vi "TCE_SaveConfiguration.vi"(0 "input cluster":T1={"Core"={"Current VI Reference"=refnum, "Close Panel on Exit?"=FALSE}, "Image Out"=refnum, "State"=0, "Points"={"Top Left"={"X"=0.0, "Y"=0.0}, "Top Right"={"X"=0.0, "Y"=0.0}, "Bottom Left"={"X"=0.0, "Y"=0.0}, "Bottom Right"={"X"=0.0, "Y"=0.0}, "x space 2"=0.0, "y space 2"=0.0, "x_space"=0.0, "y_space"=0.0, "Pixels"=[], "Fixpoint"={"X"=0.0, "Y"=0.0}}, "img_array"=[], "Temps"=[], "Temps_Array"=[], "Scan Area"=0.0, "Fixpoint Area"=0.0, "Config"={"Freezing"={"Cutoff"=2.0, "EndIndex"=2}}, "PCR Size"=0, "ImageCount"=0, "ShowGradient"=FALSE} {"Points"."Bottom Right"."Y" format="%.2f"; "Points"."Bottom Right"."X" format="%.2f"; "Points"."Top Left"."Y" format="%.2f"; "Points"."Top Left"."X" format="%.2f"; "Points"."Top Right"."Y" format="%.2f"; "Points"."Top Right"."X" format="%.2f"; "Points"."Bottom Left"."Y" format="%.2f"; "Points"."Bottom Left"."X" format="%.2f"; "Points"."Fixpoint"."Y" format="%.2f"; "Points"."Fixpoint"."X" format="%.2f"}, 1 "Temps":dbl[][](graph), 2 "FreezeTemps":dbl[](array[numeric]), 3 "MeltTemps":dbl[](array[numeric]), 4 "FrozenFraction":dbl[](array[numeric]), 5 "PartitionArray":string[](array[string]), 7 "Offsets":dbl[](array[numeric]), 9 "Offset Applied?":bool) -> (14 "Save Array out":string[][](array[string]), 17 "Full Array":string[][](array[string]), 19 "Canceled":bool)   [LabVIEW 2022 SP3]
uses:
  DataCluster_TCAL.ctl
  <vilib>/vision/Image Controls.llb/IMAQ Image.ctl
  TCE_Config.ctl
panel:
  in  "Nm(T)":bool=TRUE
  in  "SaveFrozen":bool=TRUE caption="Frozen Fraction"
  in  "SaveMelt":bool=TRUE caption="Melting Point"
  in  "SaveFreeze":bool=TRUE caption="Freezing Point"
  in  "SaveTemp":bool=TRUE caption="Temperatures"
  out "Data Array":string[][](array[string])=[["Well Name", "Content", "Freeze Temp", "Melting Temp", "T0..."], ["Calibration Offset", "Not Applied", "", "", ""], ["A1", "", "", "", ""], ["B1", "", "", "", ""], ["C1", "", "", "", ""], ["D1", "", "", "", ""], ["E1", "", "", "", ""], ["F1", "", "", "", ""], ["G1", "", "", "", ""], ["H1", "", "", "", ""], ["I1", "", "", "", ""], ["J1", "", "", "", ""], ["K1", "", "", "", ""], ["L1", "", "", "", ""], ["M1", "", "", "", ""], ["N1", "", "", "", ""], ["O1", "", "", "", ""], ["P1", "", "", "", ""], ["A2", "", "", "", ""], ["B2", "", "", "", ""], ["C2", "", "", "", ""], ["D2", "", "", "", ""], ["E2", "", "", "", ""], ["F2", "", "", "", ""], ["G2", "", "", "", ""], ["H2", "", "", "", ""], ["I2", "", "", "", ""], ["J2", "", "", "", ""], ["K2", "", "", "", ""], ["L2", "", "", "", ""], ["M2", "", "", "", ""], ["N2", "", "", "", ""], ["O2", "", "", "", ""], ["P2", "", "", "", ""], ["A3", "", "", "", ""], ["B3", "", "", "", ""], ["C3", "", "", "", ""], ["D3", "", "", "", ""], ["E3", "", "", "", ""], ["F3", "", "", "", ""], ["G3", "", "", "", ""], ["H3", "", "", "", ""], ["I3", "", "", "", ""], ["J3", "", "", "", ""], ["K3", "", "", "", ""], ["L3", "", "", "", ""], ["M3", "", "", "", ""], ["N3", "", "", "", ""], ["O3", "", "", "", ""], ["P3", "", "", "", ""], ["A4", "", "", "", ""], ["B4", "", "", "", ""], ["C4", "", "", "", ""], ["D4", "", "", "", ""], ["E4", "", "", "", ""], ["F4", "", "", "", ""], ["G4", "", "", "", ""], ["H4", "", "", "", ""], ["I4", "", "", "", ""], ["J4", "", "", "", ""], ["K4", "", "", "", ""], ["L4", "", "", "", ""], ["M4", "", "", "", ""], ["N4", "", "", "", ""], ["O4", "", "", "", ""], ["P4", "", "", "", ""], ["A5", "", "", "", ""], ["B5", "", "", "", ""], ["C5", "", "", "", ""], ["D5", "", "", "", ""], ["E5", "", "", "", ""], ["F5", "", "", "", ""], ["G5", "", "", "", ""], ["H5", "", "", "", ""], ["I5", "", "", "", ""], ["J5", "", "", "", ""], ["K5", "", "", "", ""], ["L5", "", "", "", ""], ["M5", "", "", "", ""], ["N5", "", "", "", ""], ["O5", "", "", "", ""], ["P5", "", "", "", ""], ["A6", "", "", "", ""], ["B6", "", "", "", ""], ["C6", "", "", "", ""], ["D6", "", "", "", ""], ["E6", "", "", "", ""], ["F6", "", "", "", ""], ["G6", "", "", "", ""], ["H6", "", "", "", ""], ["I6", "", "", "", ""], ["J6", "", "", "", ""], ["K6", "", "", "", ""], ["L6", "", "", "", ""], ["M6", "", "", "", ""], ["N6", "", "", "", ""], ["O6", "", "", "", ""], ["P6", "", "", "", ""], ["A7", "", "", "", ""], ["B7", "", "", "", ""], ["C7", "", "", "", ""], ["D7", "", "", "", ""], ["E7", "", "", "", ""], ["F7", "", "", "", ""], ["G7", "", "", "", ""], ["H7", "", "", "", ""], ["I7", "", "", "", ""], ["J7", "", "", "", ""], ["K7", "", "", "", ""], ["L7", "", "", "", ""], ["M7", "", "", "", ""], ["N7", "", "", "", ""], ["O7", "", "", "", ""], ["P7", "", "", "", ""], ["A8", "", "", "", ""], ["B8", "", "", "", ""], ["C8", "", "", "", ""], ["D8", "", "", "", ""], ["E8", "", "", "", ""], ["F8", "", "", "", ""], ["G8", "", "", "", ""], ["H8", "", "", "", ""], ["I8", "", "", "", ""], ["J8", "", "", "", ""], ["K8", "", "", "", ""], ["L8", "", "", "", ""], ["M8", "", "", "", ""], ["N8", "", "", "", ""], ["O8", "", "", "", ""], ["P8", "", "", "", ""], ["A9", "", "", "", ""], ["B9", "", "", "", ""], ["C9", "", "", "", ""], ["D9", "", "", "", ""], ["E9", "", "", "", ""], ["F9", "", "", "", ""], ["G9", "", "", "", ""], ["H9", "", "", "", ""], ["I9", "", "", "", ""], ["J9", "", "", "", ""], ["K9", "", "", "", ""], ["L9", "", "", "", ""], ["M9", "", "", "", ""], ["N9", "", "", "", ""], ["O9", "", "", "", ""], ["P9", "", "", "", ""], ["A10", "", "", "", ""], ["B10", "", "", "", ""], ["C10", "", "", "", ""], ["D10", "", "", "", ""], ["E10", "", "", "", ""], ["F10", "", "", "", ""], ["G10", "", "", "", ""], ["H10", "", "", "", ""], ["I10", "", "", "", ""], ["J10", "", "", "", ""], ["K10", "", "", "", ""], ["L10", "", "", "", ""], ["M10", "", "", "", ""], ["N10", "", "", "", ""], ["O10", "", "", "", ""], ["P10", "", "", "", ""], ["A11", "", "", "", ""], ["B11", "", "", "", ""], ["C11", "", "", "", ""], ["D11", "", "", "", ""], ["E11", "", "", "", ""], ["F11", "", "", "", ""], ["G11", "", "", "", ""], ["H11", "", "", "", ""], ["I11", "", "", "", ""], ["J11", "", "", "", ""], ["K11", "", "", "", ""], ["L11", "", "", "", ""], ["M11", "", "", "", ""], ["N11", "", "", "", ""], ["O11", "", "", "", ""], ["P11", "", "", "", ""], ["A12", "", "", "", ""], ["B12", "", "", "", ""], ["C12", "", "", "", ""], ["D12", "", "", "", ""], ["E12", "", "", "", ""], ["F12", "", "", "", ""], ["G12", "", "", "", ""], ["H12", "", "", "", ""], ["I12", "", "", "", ""], ["J12", "", "", "", ""], ["K12", "", "", "", ""], ["L12", "", "", "", ""], ["M12", "", "", "", ""], ["N12", "", "", "", ""], ["O12", "", "", "", ""], ["P12", "", "", "", ""], ["A13", "", "", "", ""], ["B13", "", "", "", ""], ["C13", "", "", "", ""], ["D13", "", "", "", ""], ["E13", "", "", "", ""], ["F13", "", "", "", ""], ["G13", "", "", "", ""], ["H13", "", "", "", ""], ["I13", "", "", "", ""], ["J13", "", "", "", ""], ["K13", "", "", "", ""], ["L13", "", "", "", ""], ["M13", "", "", "", ""], ["N13", "", "", "", ""], ["O13", "", "", "", ""], ["P13", "", "", "", ""], ["A14", "", "", "", ""], ["B14", "", "", "", ""], ["C14", "", "", "", ""], ["D14", "", "", "", ""], ["E14", "", "", "", ""], ["F14", "", "", "", ""], ["G14", "", "", "", ""], ["H14", "", "", "", ""], ["I14", "", "", "", ""], ["J14", "", "", "", ""], ["K14", "", "", "", ""], ["L14", "", "", "", ""], ["M14", "", "", "", ""], ["N14", "", "", "", ""], ["O14", "", "", "", ""], ["P14", "", "", "", ""], ["A15", "", "", "", ""], ["B15", "", "", "", ""], ["C15", "", "", "", ""], ["D15", "", "", "", ""], ["E15", "", "", "", ""], ["F15", "", "", "", ""], ["G15", "", "", "", ""], ["H15", "", "", "", ""], ["I15", "", "", "", ""], ["J15", "", "", "", ""], ["K15", "", "", "", ""], ["L15", "", "", "", ""], ["M15", "", "", "", ""], ["N15", "", "", "", ""], ["O15", "", "", "", ""], ["P15", "", "", "", ""], ["A16", "", "", "", ""], ["B16", "", "", "", ""], ["C16", "", "", "", ""], ["D16", "", "", "", ""], ["E16", "", "", "", ""], ["F16", "", "", "", ""], ["G16", "", "", "", ""], ["H16", "", "", "", ""], ["I16", "", "", "", ""], ["J16", "", "", "", ""], ["K16", "", "", "", ""], ["L16", "", "", "", ""], ["M16", "", "", "", ""], ["N16", "", "", "", ""], ["O16", "", "", "", ""], ["P16", "", "", "", ""], ["A17", "", "", "", ""], ["B17", "", "", "", ""], ["C17", "", "", "", ""], ["D17", "", "", "", ""], ["E17", "", "", "", ""], ["F17", "", "", "", ""], ["G17", "", "", "", ""], ["H17", "", "", "", ""], ["I17", "", "", "", ""], ["J17", "", "", "", ""], ["K17", "", "", "", ""], ["L17", "", "", "", ""], ["M17", "", "", "", ""], ["N17", "", "", "", ""], ["O17", "", "", "", ""], ["P17", "", "", "", ""], ["A18", "", "", "", ""], ["B18", "", "", "", ""], ["C18", "", "", "", ""], ["D18", "", "", "", ""], ["E18", "", "", "", ""], ["F18", "", "", "", ""], ["G18", "", "", "", ""], ["H18", "", "", "", ""], ["I18", "", "", "", ""], ["J18", "", "", "", ""], ["K18", "", "", "", ""], ["L18", "", "", "", ""], ["M18", "", "", "", ""], ["N18", "", "", "", ""], ["O18", "", "", "", ""], ["P18", "", "", "", ""], ["A19", "", "", "", ""], ["B19", "", "", "", ""], ["C19", "", "", "", ""], ["D19", "", "", "", ""], ["E19", "", "", "", ""], ["F19", "", "", "", ""], ["G19", "", "", "", ""], ["H19", "", "", "", ""], ["I19", "", "", "", ""], ["J19", "", "", "", ""], ["K19", "", "", "", ""], ["L19", "", "", "", ""], ["M19", "", "", "", ""], ["N19", "", "", "", ""], ["O19", "", "", "", ""], ["P19", "", "", "", ""], ["A20", "", "", "", ""], ["B20", "", "", "", ""], ["C20", "", "", "", ""], ["D20", "", "", "", ""], ["E20", "", "", "", ""], ["F20", "", "", "", ""], ["G20", "", "", "", ""], ["H20", "", "", "", ""], ["I20", "", "", "", ""], ["J20", "", "", "", ""], ["K20", "", "", "", ""], ["L20", "", "", "", ""], ["M20", "", "", "", ""], ["N20", "", "", "", ""], ["O20", "", "", "", ""], ["P20", "", "", "", ""], ["A21", "", "", "", ""], ["B21", "", "", "", ""], ["C21", "", "", "", ""], ["D21", "", "", "", ""], ["E21", "", "", "", ""], ["F21", "", "", "", ""], ["G21", "", "", "", ""], ["H21", "", "", "", ""], ["I21", "", "", "", ""], ["J21", "", "", "", ""], ["K21", "", "", "", ""], ["L21", "", "", "", ""], ["M21", "", "", "", ""], ["N21", "", "", "", ""], ["O21", "", "", "", ""], ["P21", "", "", "", ""], ["A22", "", "", "", ""], ["B22", "", "", "", ""], ["C22", "", "", "", ""], ["D22", "", "", "", ""], ["E22", "", "", "", ""], ["F22", "", "", "", ""], ["G22", "", "", "", ""], ["H22", "", "", "", ""], ["I22", "", "", "", ""], ["J22", "", "", "", ""], ["K22", "", "", "", ""], ["L22", "", "", "", ""], ["M22", "", "", "", ""], ["N22", "", "", "", ""], ["O22", "", "", "", ""], ["P22", "", "", "", ""], ["A23", "", "", "", ""], ["B23", "", "", "", ""], ["C23", "", "", "", ""], ["D23", "", "", "", ""], ["E23", "", "", "", ""], ["F23", "", "", "", ""], ["G23", "", "", "", ""], ["H23", "", "", "", ""], ["I23", "", "", "", ""], ["J23", "", "", "", ""], ["K23", "", "", "", ""], ["L23", "", "", "", ""], ["M23", "", "", "", ""], ["N23", "", "", "", ""], ["O23", "", "", "", ""], ["P23", "", "", "", ""], ["A24", "", "", "", ""], ["B24", "", "", "", ""], ["C24", "", "", "", ""], ["D24", "", "", "", ""], ["E24", "", "", "", ""], ["F24", "", "", "", ""], ["G24", "", "", "", ""], ["H24", "", "", "", ""], ["I24", "", "", "", ""], ["J24", "", "", "", ""], ["K24", "", "", "", ""], ["L24", "", "", "", ""], ["M24", "", "", "", ""], ["N24", "", "", "", ""], ["O24", "", "", "", ""], ["P24", "", "", "", ""]]
  in  "Cancel":bool
  in  "OK":bool
  # "Settings"
  # "File Preview"
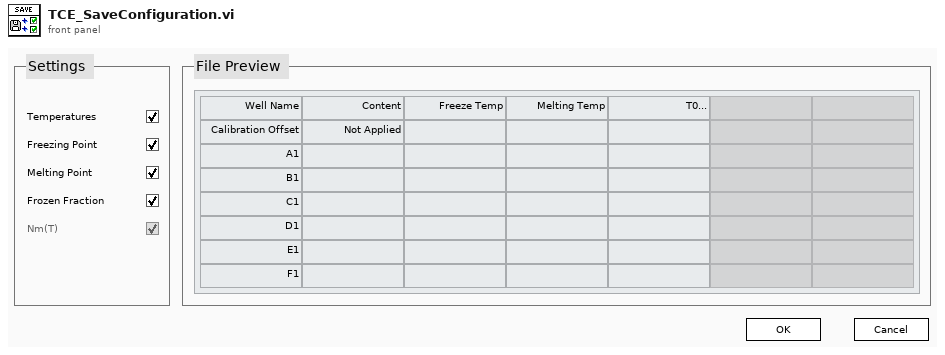
[diagram p1: front panel]
types:
  T1 = typedef "DataCluster_TCAL.ctl" = cluster{"Core":cluster{"Current VI Reference":refnum<vi>, "Close Panel on Exit?":bool}, "Image Out":T2, "State":i32, "Points":cluster{"Top Left":T3, "Top Right":T3, "Bottom Left":T3, "Bottom Right":T3, "x space 2":dbl, "y space 2":sgl, "x_space":sgl, "y_space":sgl, "Pixels":cluster{"X":i32, "Y":i32}[][], "Fixpoint":T3}, "img_array":T2[], "Temps":dbl[], "Temps_Array":dbl[][], "Scan Area":dbl, "Fixpoint Area":dbl, "Config":T4, "PCR Size":u16, "ImageCount":i32, "ShowGradient":bool}
  T2 = typedef "IMAQ Image.ctl" = refnum<image>
  T3 = typedef "IMAQ Point" = cluster{"X":sgl, "Y":sgl}
  T4 = typedef "TCE_Config.ctl" = cluster{"Freezing":cluster{"Cutoff":dbl, "EndIndex":i32}}
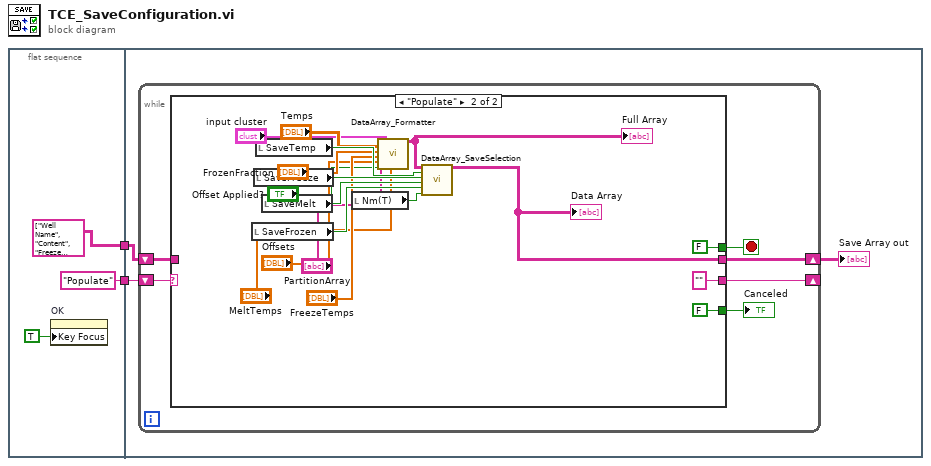
[diagram p0: block diagram]
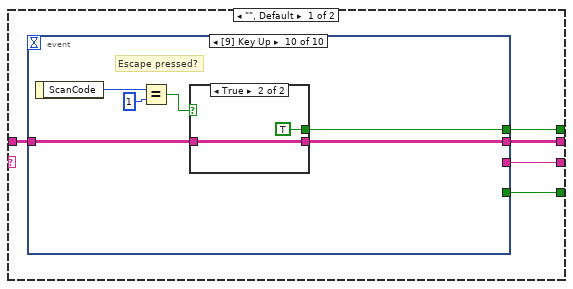
[diagram p2: hidden frame]
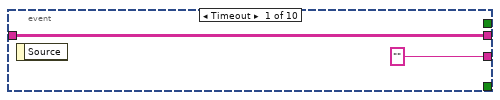
[diagram p3: hidden frame]
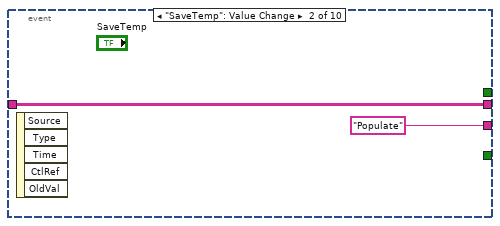
[diagram p4: hidden frame]
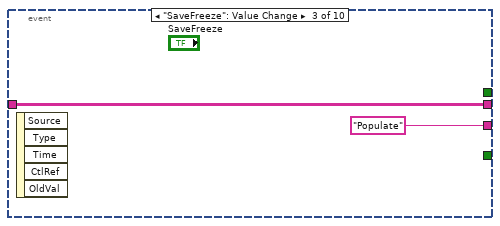
[diagram p5: hidden frame]
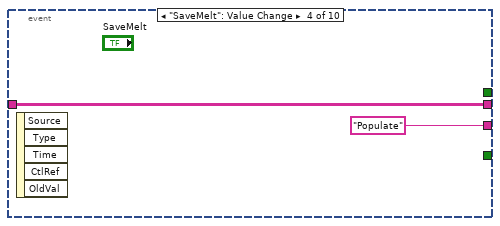
[diagram p6: hidden frame]
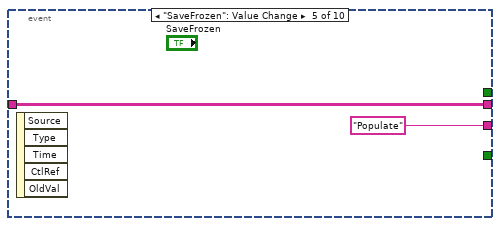
[diagram p7: hidden frame]
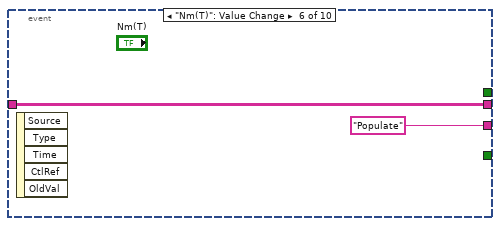
[diagram p8: hidden frame]
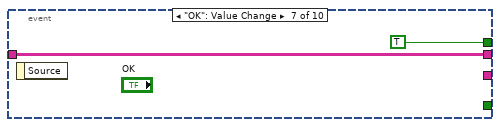
[diagram p9: hidden frame]
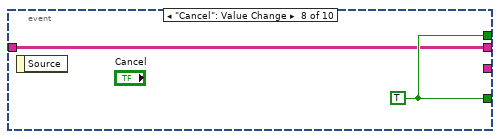
[diagram p10: hidden frame]
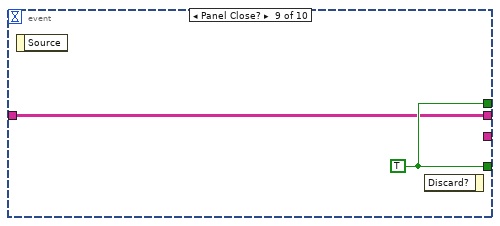
[diagram p11: hidden frame]
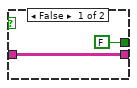
[diagram p12: hidden frame]
diagram:
  n1 = flat-sequence {
    tunnel: [string[][] [["Well Name", "Content", "Freeze Temp", "Melting Temp", "T0..."], ["Calibration Offset", "Not Applied", "", "", ""], ["A1", "", "", "", ""], ["B1", "", "", "", ""], ["C1", "", "", "", ""], ["D1", "", "", "", ""], ["E1", "", "", "", ""], ["F1", "", "", "", ""], ["G1", "", "", "", ""], ["H1", "", "", "", ""], ["I1", "", "", "", ""], ["J1", "", "", "", ""], ["K1", "", "", "", ""], ["L1", "", "", "", ""], ["M1", "", "", "", ""], ["N1", "", "", "", ""], ["O1", "", "", "", ""], ["P1", "", "", "", ""], ["A2", "", "", "", ""], ["B2", "", "", "", ""], ["C2", "", "", "", ""], ["D2", "", "", "", ""], ["E2", "", "", "", ""], ["F2", "", "", "", ""], ["G2", "", "", "", ""], ["H2", "", "", "", ""], ["I2", "", "", "", ""], ["J2", "", "", "", ""], ["K2", "", "", "", ""], ["L2", "", "", "", ""], ["M2", "", "", "", ""], ["N2", "", "", "", ""], ["O2", "", "", "", ""], ["P2", "", "", "", ""], ["A3", "", "", "", ""], ["B3", "", "", "", ""], ["C3", "", "", "", ""], ["D3", "", "", "", ""], ["E3", "", "", "", ""], ["F3", "", "", "", ""], ["G3", "", "", "", ""], ["H3", "", "", "", ""], ["I3", "", "", "", ""], ["J3", "", "", "", ""], ["K3", "", "", "", ""], ["L3", "", "", "", ""], ["M3", "", "", "", ""], ["N3", "", "", "", ""], ["O3", "", "", "", ""], ["P3", "", "", "", ""], ["A4", "", "", "", ""], ["B4", "", "", "", ""], ["C4", "", "", "", ""], ["D4", "", "", "", ""], ["E4", "", "", "", ""], ["F4", "", "", "", ""], ["G4", "", "", "", ""], ["H4", "", "", "", ""], ["I4", "", "", "", ""], ["J4", "", "", "", ""], ["K4", "", "", "", ""], ["L4", "", "", "", ""], ["M4", "", "", "", ""], ["N4", "", "", "", ""], ["O4", "", "", "", ""], ["P4", "", "", "", ""], ["A5", "", "", "", ""], ["B5", "", "", "", ""], ["C5", "", "", "", ""], ["D5", "", "", "", ""], ["E5", "", "", "", ""], ["F5", "", "", "", ""], ["G5", "", "", "", ""], ["H5", "", "", "", ""], ["I5", "", "", "", ""], ["J5", "", "", "", ""], ["K5", "", "", "", ""], ["L5", "", "", "", ""], ["M5", "", "", "", ""], ["N5", "", "", "", ""], ["O5", "", "", "", ""], ["P5", "", "", "", ""], ["A6", "", "", "", ""], ["B6", "", "", "", ""], ["C6", "", "", "", ""], ["D6", "", "", "", ""], ["E6", "", "", "", ""], ["F6", "", "", "", ""], ["G6", "", "", "", ""], ["H6", "", "", "", ""], ["I6", "", "", "", ""], ["J6", "", "", "", ""], ["K6", "", "", "", ""], ["L6", "", "", "", ""], ["M6", "", "", "", ""], ["N6", "", "", "", ""], ["O6", "", "", "", ""], ["P6", "", "", "", ""], ["A7", "", "", "", ""], ["B7", "", "", "", ""], ["C7", "", "", "", ""], ["D7", "", "", "", ""], ["E7", "", "", "", ""], ["F7", "", "", "", ""], ["G7", "", "", "", ""], ["H7", "", "", "", ""], ["I7", "", "", "", ""], ["J7", "", "", "", ""], ["K7", "", "", "", ""], ["L7", "", "", "", ""], ["M7", "", "", "", ""], ["N7", "", "", "", ""], ["O7", "", "", "", ""], ["P7", "", "", "", ""], ["A8", "", "", "", ""], ["B8", "", "", "", ""], ["C8", "", "", "", ""], ["D8", "", "", "", ""], ["E8", "", "", "", ""], ["F8", "", "", "", ""], ["G8", "", "", "", ""], ["H8", "", "", "", ""], ["I8", "", "", "", ""], ["J8", "", "", "", ""], ["K8", "", "", "", ""], ["L8", "", "", "", ""], ["M8", "", "", "", ""], ["N8", "", "", "", ""], ["O8", "", "", "", ""], ["P8", "", "", "", ""], ["A9", "", "", "", ""], ["B9", "", "", "", ""], ["C9", "", "", "", ""], ["D9", "", "", "", ""], ["E9", "", "", "", ""], ["F9", "", "", "", ""], ["G9", "", "", "", ""], ["H9", "", "", "", ""], ["I9", "", "", "", ""], ["J9", "", "", "", ""], ["K9", "", "", "", ""], ["L9", "", "", "", ""], ["M9", "", "", "", ""], ["N9", "", "", "", ""], ["O9", "", "", "", ""], ["P9", "", "", "", ""], ["A10", "", "", "", ""], ["B10", "", "", "", ""], ["C10", "", "", "", ""], ["D10", "", "", "", ""], ["E10", "", "", "", ""], ["F10", "", "", "", ""], ["G10", "", "", "", ""], ["H10", "", "", "", ""], ["I10", "", "", "", ""], ["J10", "", "", "", ""], ["K10", "", "", "", ""], ["L10", "", "", "", ""], ["M10", "", "", "", ""], ["N10", "", "", "", ""], ["O10", "", "", "", ""], ["P10", "", "", "", ""], ["A11", "", "", "", ""], ["B11", "", "", "", ""], ["C11", "", "", "", ""], ["D11", "", "", "", ""], ["E11", "", "", "", ""], ["F11", "", "", "", ""], ["G11", "", "", "", ""], ["H11", "", "", "", ""], ["I11", "", "", "", ""], ["J11", "", "", "", ""], ["K11", "", "", "", ""], ["L11", "", "", "", ""], ["M11", "", "", "", ""], ["N11", "", "", "", ""], ["O11", "", "", "", ""], ["P11", "", "", "", ""], ["A12", "", "", "", ""], ["B12", "", "", "", ""], ["C12", "", "", "", ""], ["D12", "", "", "", ""], ["E12", "", "", "", ""], ["F12", "", "", "", ""], ["G12", "", "", "", ""], ["H12", "", "", "", ""], ["I12", "", "", "", ""], ["J12", "", "", "", ""], ["K12", "", "", "", ""], ["L12", "", "", "", ""], ["M12", "", "", "", ""], ["N12", "", "", "", ""], ["O12", "", "", "", ""], ["P12", "", "", "", ""], ["A13", "", "", "", ""], ["B13", "", "", "", ""], ["C13", "", "", "", ""], ["D13", "", "", "", ""], ["E13", "", "", "", ""], ["F13", "", "", "", ""], ["G13", "", "", "", ""], ["H13", "", "", "", ""], ["I13", "", "", "", ""], ["J13", "", "", "", ""], ["K13", "", "", "", ""], ["L13", "", "", "", ""], ["M13", "", "", "", ""], ["N13", "", "", "", ""], ["O13", "", "", "", ""], ["P13", "", "", "", ""], ["A14", "", "", "", ""], ["B14", "", "", "", ""], ["C14", "", "", "", ""], ["D14", "", "", "", ""], ["E14", "", "", "", ""], ["F14", "", "", "", ""], ["G14", "", "", "", ""], ["H14", "", "", "", ""], ["I14", "", "", "", ""], ["J14", "", "", "", ""], ["K14", "", "", "", ""], ["L14", "", "", "", ""], ["M14", "", "", "", ""], ["N14", "", "", "", ""], ["O14", "", "", "", ""], ["P14", "", "", "", ""], ["A15", "", "", "", ""], ["B15", "", "", "", ""], ["C15", "", "", "", ""], ["D15", "", "", "", ""], ["E15", "", "", "", ""], ["F15", "", "", "", ""], ["G15", "", "", "", ""], ["H15", "", "", "", ""], ["I15", "", "", "", ""], ["J15", "", "", "", ""], ["K15", "", "", "", ""], ["L15", "", "", "", ""], ["M15", "", "", "", ""], ["N15", "", "", "", ""], ["O15", "", "", "", ""], ["P15", "", "", "", ""], ["A16", "", "", "", ""], ["B16", "", "", "", ""], ["C16", "", "", "", ""], ["D16", "", "", "", ""], ["E16", "", "", "", ""], ["F16", "", "", "", ""], ["G16", "", "", "", ""], ["H16", "", "", "", ""], ["I16", "", "", "", ""], ["J16", "", "", "", ""], ["K16", "", "", "", ""], ["L16", "", "", "", ""], ["M16", "", "", "", ""], ["N16", "", "", "", ""], ["O16", "", "", "", ""], ["P16", "", "", "", ""], ["A17", "", "", "", ""], ["B17", "", "", "", ""], ["C17", "", "", "", ""], ["D17", "", "", "", ""], ["E17", "", "", "", ""], ["F17", "", "", "", ""], ["G17", "", "", "", ""], ["H17", "", "", "", ""], ["I17", "", "", "", ""], ["J17", "", "", "", ""], ["K17", "", "", "", ""], ["L17", "", "", "", ""], ["M17", "", "", "", ""], ["N17", "", "", "", ""], ["O17", "", "", "", ""], ["P17", "", "", "", ""], ["A18", "", "", "", ""], ["B18", "", "", "", ""], ["C18", "", "", "", ""], ["D18", "", "", "", ""], ["E18", "", "", "", ""], ["F18", "", "", "", ""], ["G18", "", "", "", ""], ["H18", "", "", "", ""], ["I18", "", "", "", ""], ["J18", "", "", "", ""], ["K18", "", "", "", ""], ["L18", "", "", "", ""], ["M18", "", "", "", ""], ["N18", "", "", "", ""], ["O18", "", "", "", ""], ["P18", "", "", "", ""], ["A19", "", "", "", ""], ["B19", "", "", "", ""], ["C19", "", "", "", ""], ["D19", "", "", "", ""], ["E19", "", "", "", ""], ["F19", "", "", "", ""], ["G19", "", "", "", ""], ["H19", "", "", "", ""], ["I19", "", "", "", ""], ["J19", "", "", "", ""], ["K19", "", "", "", ""], ["L19", "", "", "", ""], ["M19", "", "", "", ""], ["N19", "", "", "", ""], ["O19", "", "", "", ""], ["P19", "", "", "", ""], ["A20", "", "", "", ""], ["B20", "", "", "", ""], ["C20", "", "", "", ""], ["D20", "", "", "", ""], ["E20", "", "", "", ""], ["F20", "", "", "", ""], ["G20", "", "", "", ""], ["H20", "", "", "", ""], ["I20", "", "", "", ""], ["J20", "", "", "", ""], ["K20", "", "", "", ""], ["L20", "", "", "", ""], ["M20", "", "", "", ""], ["N20", "", "", "", ""], ["O20", "", "", "", ""], ["P20", "", "", "", ""], ["A21", "", "", "", ""], ["B21", "", "", "", ""], ["C21", "", "", "", ""], ["D21", "", "", "", ""], ["E21", "", "", "", ""], ["F21", "", "", "", ""], ["G21", "", "", "", ""], ["H21", "", "", "", ""], ["I21", "", "", "", ""], ["J21", "", "", "", ""], ["K21", "", "", "", ""], ["L21", "", "", "", ""], ["M21", "", "", "", ""], ["N21", "", "", "", ""], ["O21", "", "", "", ""], ["P21", "", "", "", ""], ["A22", "", "", "", ""], ["B22", "", "", "", ""], ["C22", "", "", "", ""], ["D22", "", "", "", ""], ["E22", "", "", "", ""], ["F22", "", "", "", ""], ["G22", "", "", "", ""], ["H22", "", "", "", ""], ["I22", "", "", "", ""], ["J22", "", "", "", ""], ["K22", "", "", "", ""], ["L22", "", "", "", ""], ["M22", "", "", "", ""], ["N22", "", "", "", ""], ["O22", "", "", "", ""], ["P22", "", "", "", ""], ["A23", "", "", "", ""], ["B23", "", "", "", ""], ["C23", "", "", "", ""], ["D23", "", "", "", ""], ["E23", "", "", "", ""], ["F23", "", "", "", ""], ["G23", "", "", "", ""], ["H23", "", "", "", ""], ["I23", "", "", "", ""], ["J23", "", "", "", ""], ["K23", "", "", "", ""], ["L23", "", "", "", ""], ["M23", "", "", "", ""], ["N23", "", "", "", ""], ["O23", "", "", "", ""], ["P23", "", "", "", ""], ["A24", "", "", "", ""], ["B24", "", "", "", ""], ["C24", "", "", "", ""], ["D24", "", "", "", ""], ["E24", "", "", "", ""], ["F24", "", "", "", ""], ["G24", "", "", "", ""], ["H24", "", "", "", ""], ["I24", "", "", "", ""], ["J24", "", "", "", ""], ["K24", "", "", "", ""], ["L24", "", "", "", ""], ["M24", "", "", "", ""], ["N24", "", "", "", ""], ["O24", "", "", "", ""], ["P24", "", "", "", ""]] ("Data Array out")] -> w2
    tunnel: ["Populate"] -> w1
    tunnel: w2 -> [w8]
    tunnel: w1 -> [w7]
    frame #0 {
      n2 = property on="OK" class="Bool"("Key Focus"=TRUE) -> ()  [unwired: 2 in, 2 out]
    }
    frame #1 {
      n3 = while {
        shift-right: [w14] -> w6
        shift-left: w8 -> [w13]
        shift-right: [w9] -> _
        shift-left: w7 -> [w10]
        stop <- w12 stop-if-true
        n4 = case shown="\"Populate\"" w10 {
          tunnel: [w19 w48] -> w14
          tunnel: w13 -> [w18 _]
          tunnel: [w17 FALSE] -> w12
          tunnel: [w16 FALSE] -> w11
          tunnel: [w15 ""] -> w9
          frame "", Default {
            n5 = event shown="[9] Key Up" {
              selector: _ -> [_ _ _ _ _ _ _ _ _ _]
              dyn-events: _ -> [_ _ _ _ _ _ _ _ _ _]
              timeout: _ -> [_ _ _ _ _ _ _ _ _ _]
              tunnel: w18 -> [w20 w22 w24 w26 w28 w30 w33 w34 w36 w38]
              tunnel: [w20 w22 w24 w26 w28 w30 w33 w34 w36 w39] -> w19
              tunnel: [_ _ _ _ _ _ TRUE w35 w37 w43] -> w17
              tunnel: [_ _ _ _ _ _ _ w35 w37 _] -> w16
              tunnel: ["" "Populate" "Populate" "Populate" "Populate" "Populate" _ _ _ _] -> w15
              event Timeout {
                n6 = event-data() -> ()  [unwired: 1 in, 1 out]
              }
              event "SaveTemp": Value Change {
                n7 = event-data() -> ()  [unwired: 1 in, 5 out]
              }
              event "SaveFreeze": Value Change {
                n8 = event-data() -> ()  [unwired: 1 in, 5 out]
              }
              event "SaveMelt": Value Change {
                n9 = event-data() -> ()  [unwired: 1 in, 5 out]
              }
              event "SaveFrozen": Value Change {
                n10 = event-data() -> ()  [unwired: 1 in, 5 out]
              }
              event "Nm(T)": Value Change {
                n11 = event-data() -> ()  [unwired: 1 in, 5 out]
              }
              event "OK": Value Change {
                n12 = event-data() -> ()  [unwired: 1 in, 1 out]
              }
              event "Cancel": Value Change {
                w35 = TRUE
                n13 = event-data() -> ()  [unwired: 1 in, 1 out]
              }
              event Panel Close? {
                w37 = TRUE
                n14 = event-data() -> ()  [unwired: 1 in, 1 out]
                n15 = event-data() -> ()  [unwired: 2 in, 1 out]
              }
              event Key Up {
                # "Escape pressed?"
                n16 = event-data() -> ("ScanCode"=w42:i16)  [unwired: 1 in]
                n17 = Equal?(x=w42, y=i16 1) -> (x = y?=w40:bool)
                n18 = case shown="True" w40 {
                  tunnel: [FALSE TRUE] -> w43
                  tunnel: [w45 w46] -> w39
                  tunnel: w38 -> [w45 w46]
                  frame False {
                  }
                  frame True {
                  }
                }
              }
            }
          }
          frame "Populate" {
            n19 = local read "SaveFrozen"() -> (w59:bool)
            n20 = local read "SaveFreeze"() -> (w57:bool)
            n21 = local read "SaveTemp"() -> (w61:bool)
            n22 = local read "SaveMelt"() -> (w58:bool)
            n23 = local read "Nm(T)"() -> (w60:bool)
            n24 = call "DataArray_Formatter.vi"("PartitionArray"="PartitionArray", "Temps"="Temps", "FrozenFraction"="FrozenFraction", "FreezeTemps"="FreezeTemps", "Offsets"="Offsets", "Offset Applied?"="Offset Applied?", "input cluster"="input cluster", "MeltTemps"="MeltTemps") -> ("Data Array"=w62:string[][])  [unwired: 11 in]
            "Full Array" <- w62
            n25 = call "DataArray_SaveSelection.vi"("Data Array"=w62, "SaveTemp"=w61, "SaveFreeze"=w57, "SaveMelt"=w58, "SaveFrozen"=w59, "Nm(T)"=w60) -> ("Data Array out"=w48:string[][])  [unwired: 13 in]
            "Data Array" <- w48
          }
        }
        "Canceled" <- w11
      }
      "Save Array out" <- w6
    }
  }
